vi "nanocal frontend server 18.vi"() -> ()   [LabVIEW 2018]
uses:
  nanocal/Nanocalorimetry/data/NanoCalLib.lvlibp/NanoReadings/NanoReadings_Parameters_TypeDef.ctl
  nanocal/Nanocalorimetry/data/NanoCalLib.lvlibp/NanoReadings/NanoReadings_Power.ctl
  nanocal/Nanocalorimetry/data/NanoCalLib.lvlibp/NanoReadings/NanoReadings_CandK.ctl
  nanocal/Nanocalorimetry/data/NanoCalLib.lvlibp/NanoReadings/NanoReadings_IandV.ctl
  nanocal/Nanocalorimetry/data/NanoCalLib.lvlibp/NanoReadings/NanoReadings_TdcTac.ctl
  nanocal/Nanocalorimetry/data/NanoCalLib.lvlibp/NanoReadings/NanoReadings_Phases.ctl
  nanocal/Nanocalorimetry/data/NanoCalLib.lvlibp/NanoReadings/NanoReadings_Frequencies.ctl
  nanocal/Nanocalorimetry/data/NanoCalLib.lvlibp/NanoReadings/NanoReadings_FirstHarmonic.ctl
  nanocal/Nanocalorimetry/data/NanoCalLib.lvlibp/NanoReadings/NanoReadings_Output.ctl
  nanocal/Nanocalorimetry/data/NanoCalLib.lvlibp/NanoReadings/NanoReadings_MagneticFieldEtc.ctl
  nanocal/Nanocalorimetry/data/NanoCalLib.lvlibp/NanoReadings/NanoReadings_Calibration.ctl
  nanocal/Nanocalorimetry/data/NanoCalLib.lvlibp/NanoReadings/NanoReadings_CTetc.ctl
  nanocal/Nanocalorimetry/data/NanoCalLib.lvlibp/NanoReadings/NanoReadings_2ndHarmonic.ctl
  nanocal/Nanocalorimetry/data/NanoCalLib.lvlibp/NanoReadings/NanoReadings_Resistance.ctl
  nanocal/Nanocalorimetry/data/NanoCalLib.lvlibp/NanoReadings/NanoReadings_TimeEtc.ctl
  frontend -- data type.ctl
  nanocal/Nanocalorimetry/data/NanoCalLib.lvlibp
  nanocal/Nanocalorimetry/data/NanoCalLib.lvlibp/NanoReadings/NanoReadings.lvlib
panel:
  in  "Latest data 2":T1={"Power"={"PHs (W)"=0.0, "PHr (W)"=0.0, "Ps,dc (W)"=0.0, "Pr,dc (W)"=0.0, "PHs,dc (W)"=0.0, "PHr,dc (W)"=0.0, "Ps,ac (W)"=0.0, "Pr,ac (W)"=0.0, "PHs/PHr"=0.0, "Poffs (W)"=0.0, "Ps total (W)"=0.0, "Pr total (W)"=0.0, "Ps-Pr total (W)"=0.0, "Ps,offs (W)"=0.0}, "C and K"={"Cs (J/K)"=0.0, "Ks (W/K)"=0.0, "Cr (J/K)"=0.0, "Kr (W/K)"=0.0, "Cdiff (J/K)"=0.0, "Cs-Cr (J/K)"=0.0, "Cdiff old style (J/K)"=0.0, "Cr from S,diff (J/K)"=0.0}, "IV dc"={"Is,dc (A)"=0.0, "Ir,dc (A)"=0.0, "Us,dc (V)"=0.0, "Ur,dc (V)"=0.0, "Udiff,dc (V)"=0.0, "IHs dc (A)"=0.0, "UHs dc (V)"=0.0, "IHr dc (A)"=0.0, "UHr dc (V)"=0.0, "Uoffs dc (V)"=0.0, "Ioffs dc (A)"=0.0}, "Tdc,Tac"={"Ts (K)"=0.0, "Tr (K)"=0.0, "Tdiff from Rs,Rr"=0.0, "Tdiff from Udiff (K)"=0.0, "Ts,ac (K)"=0.0, "Tr,ac (K)"=0.0, "Tdiff,ac (K)"=0.0, "Ts,ac driftcorr (K)"=0.0, "Tr,ac driftcorr (K)"=0.0, "Tr,ac from Ts,diff,ac (K)"=0.0, "T target (K)"=0.0}, "Phases"={"Phi Is (deg)"=0.0, "Phi Us (deg)"=0.0, "Phi Ir (deg)"=0.0, "Phi Ur (deg)"=0.0, "Phi Udiff (deg)"=0.0, "Phi IHs (deg)"=0.0, "Phi UHs (deg)"=0.0, "Phi IHr (deg)"=0.0, "Phi UHr (deg)"=0.0, "Phi R from S,diff (deg)"=0.0, "Phi Is 1st (deg)"=0.0, "Phi Us 1st (deg)"=0.0, "Phi Ir 1st (deg)"=0.0, "Phi Ur 1st (deg)"=0.0, "Phi Udiff 1st (deg)"=0.0, "Phi Udiff, raw (deg)"=0.0}, "f etc"={"f (Hz)"=36.0, "f therm (Hz)"=0.0, "omega (rad/s)"=0.0, "Tan Phi S/diff"=0.0, "Sin Phi"=0.0, "Cos Phi"=0.0, "f mix (Hz)"=0.0, "tau (s)"=0.0}, "IV 1st harm"={"Is,ac 1st (A)"=0.0, "Ir,ac 1st (A)"=0.0, "Us,ac 1st (V)"=0.0, "Ur,ac 1st (V)"=0.0, "Udiff,ac 1st (V)"=0.0, "IHs (A)"=0.0, "UHs (V)"=0.0, "IHr (A)"=0.0, "UHr (V)"=0.0}, "ForAveraging"={"SinTherm"=[], "CosTherm"=[], "SinHeats"=[], "CosHeats"=[]}, "Output"={"S phase (deg)"=0.0, "R phase (deg)"=0.0, "Hs ac out (Vrms)"=0.0, "Hr ac out (Vrms)"=0.0, "S Therm dc out (V)"=0.0, "R Therm dc out (V)"=0.0, "S Therm ac out (Vrms)"=0.0, "R Therm ac out (Vrms)"=0.0, "Offset dc out (V)"=0.0, "Hs dc out (V)"=0.0, "Hr dc out (V)"=0.0, "Offset ac out (Vrms)"=0.0}, "Magnetic field etc."={"H (T)"=0.0, "T probe (K)"=0.0, "Polar angle (deg)"=0.0, "Azimuthal angle (deg)"=0.0}, "Calibration"={"1+Rs/RIs factor"=0.0, "1+RIs/Rs factor"=0.0, "Rs,scaled (ohm)"=0.0, "Rr,scaled (ohm)"=0.0, "R lead S (ohm)"=0.0, "R lead R (ohm)"=0.0, "|dlnR/dlnT| S"=0.0, "|dlnR/dlnT| R"=0.0, "dTs/dt (mK/s)"=0.0, "dTr/dt (mK/s)"=0.0}, "CT etc"={"Cs/T (J/K^2)"=5.0, "Cr/T (J/K^2)"=0.0, "Cdiff/T (J/K^2)"=0.0, "(Cs-Cr)/T (J/K^2)"=0.0, "Cdiff/T old style (J/K^2)"=0.0, "Cr/T from S,diff (J/K^2)"=0.0, "Ts^2 (K^2)"=3.0, "Tr^2 (K^2)"=0.0}, "IV 2nd harm"={"Is,ac (A)"=0.0, "Ir,ac (A)"=0.0, "Us,ac (V)"=0.0, "Ur,ac (V)"=0.0, "Udiff,ac (V)"=0.0}, "Resistance"={"RHs (ohm)"=0.0, "RHr (ohm)"=0.0, "Rs (ohm)"=0.0, "Rr (ohm)"=0.0, "RHs,dc (ohm)"=0.0, "RHr,dc (ohm)"=0.0, "Rs,ac (ohm)"=0.0, "Rr,ac (ohm)"=0.0, "Roffs (ohm)"=0.0}, "Time etc"={"Time (s)"=0.0, "Datapoint index"=0.0, "Datapoint time (s)"=0.0}} {"Time etc"."Datapoint time (s)" format="%#_7g"; "Time etc"."Datapoint index" format="%#_7g"; "Time etc"."Time (s)" format="%#_7g"; "Resistance"."Roffs (ohm)" format="%#_7g"; "Resistance"."Rr,ac (ohm)" format="%#_7g"; "Resistance"."Rs,ac (ohm)" format="%#_7g"; "Resistance"."RHr,dc (ohm)" format="%#_7g"; "Resistance"."RHs,dc (ohm)" format="%#_7g"; "Resistance"."Rr (ohm)" format="%#_7g"; "Resistance"."Rs (ohm)" format="%#_7g"; "Resistance"."RHr (ohm)" format="%#_7g"; "Resistance"."RHs (ohm)" format="%#_7g"; "IV 2nd harm"."Udiff,ac (V)" format="%#_7g"; "IV 2nd harm"."Ur,ac (V)" format="%#_7g"; "IV 2nd harm"."Us,ac (V)" format="%#_7g"; "IV 2nd harm"."Ir,ac (A)" format="%#_7g"; "IV 2nd harm"."Is,ac (A)" format="%#_7g"; "CT etc"."Tr^2 (K^2)" format="%#_7g"; "CT etc"."Ts^2 (K^2)" format="%#_7g"; "Calibration"."dTr/dt (mK/s)" format="%#_7g"; "Calibration"."dTs/dt (mK/s)" format="%#_7g"; "Output"."Hr dc out (V)" min=0.0 max=7.0707; "Output"."Hs dc out (V)" min=0.0 max=7.0707; "Output"."Hr ac out (Vrms)" min=0.0 max=7.0707; "Output"."Hs ac out (Vrms)" min=0.0 max=7.0707; "Output"."R phase (deg)" format="%#_7g"; "Output"."S phase (deg)" format="%#_7g"; "IV 1st harm"."UHr (V)" format="%#_7g"; "IV 1st harm"."IHr (A)" format="%#_7g"; "IV 1st harm"."UHs (V)" format="%#_7g"; "IV 1st harm"."IHs (A)" format="%#_7g"; "IV 1st harm"."Udiff,ac 1st (V)" format="%#_7g"; "IV 1st harm"."Ur,ac 1st (V)" format="%#_7g"; "IV 1st harm"."Us,ac 1st (V)" format="%#_7g"; "IV 1st harm"."Ir,ac 1st (A)" format="%#_7g"; "IV 1st harm"."Is,ac 1st (A)" format="%#_7g"; "f etc"."tau (s)" format="%#_7g"; "f etc"."Cos Phi" format="%#_7g"; "f etc"."Sin Phi" format="%#_7g"; "f etc"."Tan Phi S/diff" format="%#_7g"; "Phases"."Phi Udiff, raw (deg)" format="%#_7g"; "Phases"."Phi Udiff 1st (deg)" format="%#_7g"; "Phases"."Phi Ur 1st (deg)" format="%#_7g"; "Phases"."Phi Ir 1st (deg)" format="%#_7g"; "Phases"."Phi Us 1st (deg)" format="%#_7g"; "Phases"."Phi Is 1st (deg)" format="%#_7g"; "Phases"."Phi R from S,diff (deg)" format="%#_7g"; "Phases"."Phi UHr (deg)" format="%#_7g"; "Phases"."Phi IHr (deg)" format="%#_7g"; "Phases"."Phi UHs (deg)" format="%#_7g"; "Phases"."Phi IHs (deg)" format="%#_7g"; "Phases"."Phi Udiff (deg)" format="%#_7g"; "Phases"."Phi Ur (deg)" format="%#_7g"; "Phases"."Phi Ir (deg)" format="%#_7g"; "Phases"."Phi Us (deg)" format="%#_7g"; "Phases"."Phi Is (deg)" format="%#_7g"; "Tdc,Tac"."T target (K)" format="%#_7g"; "Tdc,Tac"."Tr,ac from Ts,diff,ac (K)" format="%#_7g"; "Tdc,Tac"."Tr,ac driftcorr (K)" format="%#_7g"; "Tdc,Tac"."Ts,ac driftcorr (K)" format="%#_7g"; "Tdc,Tac"."Tdiff,ac (K)" format="%#_7g"; "Tdc,Tac"."Tr,ac (K)" format="%#_7g"; "Tdc,Tac"."Ts,ac (K)" format="%#_7g"; "Tdc,Tac"."Tdiff from Udiff (K)" format="%#_7g"; "Tdc,Tac"."Tdiff from Rs,Rr" format="%#_7g"; "Tdc,Tac"."Tr (K)" format="%#_7g"; "Tdc,Tac"."Ts (K)" format="%#_7g"; "IV dc"."Ioffs dc (A)" format="%#_7g"; "IV dc"."Uoffs dc (V)" format="%#_7g"; "IV dc"."UHr dc (V)" format="%#_7g"; "IV dc"."IHr dc (A)" format="%#_7g"; "IV dc"."UHs dc (V)" format="%#_7g"; "IV dc"."IHs dc (A)" format="%#_7g"; "IV dc"."Udiff,dc (V)" format="%#_7g"; "IV dc"."Ur,dc (V)" format="%#_7g"; "IV dc"."Us,dc (V)" format="%#_7g"; "IV dc"."Ir,dc (A)" format="%#_7g"; "IV dc"."Is,dc (A)" format="%#_7g"; "Power"."Ps,offs (W)" format="%#_7g"; "Power"."Ps-Pr total (W)" format="%#_7g"; "Power"."Pr total (W)" format="%#_7g"; "Power"."Ps total (W)" format="%#_7g"; "Power"."Poffs (W)" format="%#_7g"; "Power"."PHs/PHr" format="%#_7g"; "Power"."Pr,ac (W)" format="%#_7g"; "Power"."Ps,ac (W)" format="%#_7g"; "Power"."PHr,dc (W)" format="%#_7g"; "Power"."PHs,dc (W)" format="%#_7g"; "Power"."Pr,dc (W)" format="%#_7g"; "Power"."Ps,dc (W)" format="%#_7g"; "Power"."PHr (W)" format="%#_7g"; "Power"."PHs (W)" format="%#_7g"}
  out "Numeric":i32=90
  out "output cluster":T16
  in  "milliseconds to wait":u32=100
  in  "Stop":bool
  out "Latest data":T1 {"Time etc"."Datapoint time (s)" format="%#_7g"; "Time etc"."Datapoint index" format="%#_7g"; "Time etc"."Time (s)" format="%#_7g"; "Resistance"."Roffs (ohm)" format="%#_7g"; "Resistance"."Rr,ac (ohm)" format="%#_7g"; "Resistance"."Rs,ac (ohm)" format="%#_7g"; "Resistance"."RHr,dc (ohm)" format="%#_7g"; "Resistance"."RHs,dc (ohm)" format="%#_7g"; "Resistance"."Rr (ohm)" format="%#_7g"; "Resistance"."Rs (ohm)" format="%#_7g"; "Resistance"."RHr (ohm)" format="%#_7g"; "Resistance"."RHs (ohm)" format="%#_7g"; "IV 2nd harm"."Udiff,ac (V)" format="%#_7g"; "IV 2nd harm"."Ur,ac (V)" format="%#_7g"; "IV 2nd harm"."Us,ac (V)" format="%#_7g"; "IV 2nd harm"."Ir,ac (A)" format="%#_7g"; "IV 2nd harm"."Is,ac (A)" format="%#_7g"; "CT etc"."Tr^2 (K^2)" format="%#_7g"; "CT etc"."Ts^2 (K^2)" format="%#_7g"; "Calibration"."dTr/dt (mK/s)" format="%#_7g"; "Calibration"."dTs/dt (mK/s)" format="%#_7g"; "Output"."Hr dc out (V)" min=0.0 max=7.0707; "Output"."Hs dc out (V)" min=0.0 max=7.0707; "Output"."Hr ac out (Vrms)" min=0.0 max=7.0707; "Output"."Hs ac out (Vrms)" min=0.0 max=7.0707; "Output"."R phase (deg)" format="%#_7g"; "Output"."S phase (deg)" format="%#_7g"; "IV 1st harm"."UHr (V)" format="%#_7g"; "IV 1st harm"."IHr (A)" format="%#_7g"; "IV 1st harm"."UHs (V)" format="%#_7g"; "IV 1st harm"."IHs (A)" format="%#_7g"; "IV 1st harm"."Udiff,ac 1st (V)" format="%#_7g"; "IV 1st harm"."Ur,ac 1st (V)" format="%#_7g"; "IV 1st harm"."Us,ac 1st (V)" format="%#_7g"; "IV 1st harm"."Ir,ac 1st (A)" format="%#_7g"; "IV 1st harm"."Is,ac 1st (A)" format="%#_7g"; "f etc"."tau (s)" format="%#_7g"; "f etc"."Cos Phi" format="%#_7g"; "f etc"."Sin Phi" format="%#_7g"; "f etc"."Tan Phi S/diff" format="%#_7g"; "Phases"."Phi Udiff, raw (deg)" format="%#_7g"; "Phases"."Phi Udiff 1st (deg)" format="%#_7g"; "Phases"."Phi Ur 1st (deg)" format="%#_7g"; "Phases"."Phi Ir 1st (deg)" format="%#_7g"; "Phases"."Phi Us 1st (deg)" format="%#_7g"; "Phases"."Phi Is 1st (deg)" format="%#_7g"; "Phases"."Phi R from S,diff (deg)" format="%#_7g"; "Phases"."Phi UHr (deg)" format="%#_7g"; "Phases"."Phi IHr (deg)" format="%#_7g"; "Phases"."Phi UHs (deg)" format="%#_7g"; "Phases"."Phi IHs (deg)" format="%#_7g"; "Phases"."Phi Udiff (deg)" format="%#_7g"; "Phases"."Phi Ur (deg)" format="%#_7g"; "Phases"."Phi Ir (deg)" format="%#_7g"; "Phases"."Phi Us (deg)" format="%#_7g"; "Phases"."Phi Is (deg)" format="%#_7g"; "Tdc,Tac"."T target (K)" format="%#_7g"; "Tdc,Tac"."Tr,ac from Ts,diff,ac (K)" format="%#_7g"; "Tdc,Tac"."Tr,ac driftcorr (K)" format="%#_7g"; "Tdc,Tac"."Ts,ac driftcorr (K)" format="%#_7g"; "Tdc,Tac"."Tdiff,ac (K)" format="%#_7g"; "Tdc,Tac"."Tr,ac (K)" format="%#_7g"; "Tdc,Tac"."Ts,ac (K)" format="%#_7g"; "Tdc,Tac"."Tdiff from Udiff (K)" format="%#_7g"; "Tdc,Tac"."Tdiff from Rs,Rr" format="%#_7g"; "Tdc,Tac"."Tr (K)" format="%#_7g"; "Tdc,Tac"."Ts (K)" format="%#_7g"; "IV dc"."Ioffs dc (A)" format="%#_7g"; "IV dc"."Uoffs dc (V)" format="%#_7g"; "IV dc"."UHr dc (V)" format="%#_7g"; "IV dc"."IHr dc (A)" format="%#_7g"; "IV dc"."UHs dc (V)" format="%#_7g"; "IV dc"."IHs dc (A)" format="%#_7g"; "IV dc"."Udiff,dc (V)" format="%#_7g"; "IV dc"."Ur,dc (V)" format="%#_7g"; "IV dc"."Us,dc (V)" format="%#_7g"; "IV dc"."Ir,dc (A)" format="%#_7g"; "IV dc"."Is,dc (A)" format="%#_7g"; "Power"."Ps,offs (W)" format="%#_7g"; "Power"."Ps-Pr total (W)" format="%#_7g"; "Power"."Pr total (W)" format="%#_7g"; "Power"."Ps total (W)" format="%#_7g"; "Power"."Poffs (W)" format="%#_7g"; "Power"."PHs/PHr" format="%#_7g"; "Power"."Pr,ac (W)" format="%#_7g"; "Power"."Ps,ac (W)" format="%#_7g"; "Power"."PHr,dc (W)" format="%#_7g"; "Power"."PHs,dc (W)" format="%#_7g"; "Power"."Pr,dc (W)" format="%#_7g"; "Power"."Ps,dc (W)" format="%#_7g"; "Power"."PHr (W)" format="%#_7g"; "Power"."PHs (W)" format="%#_7g"}
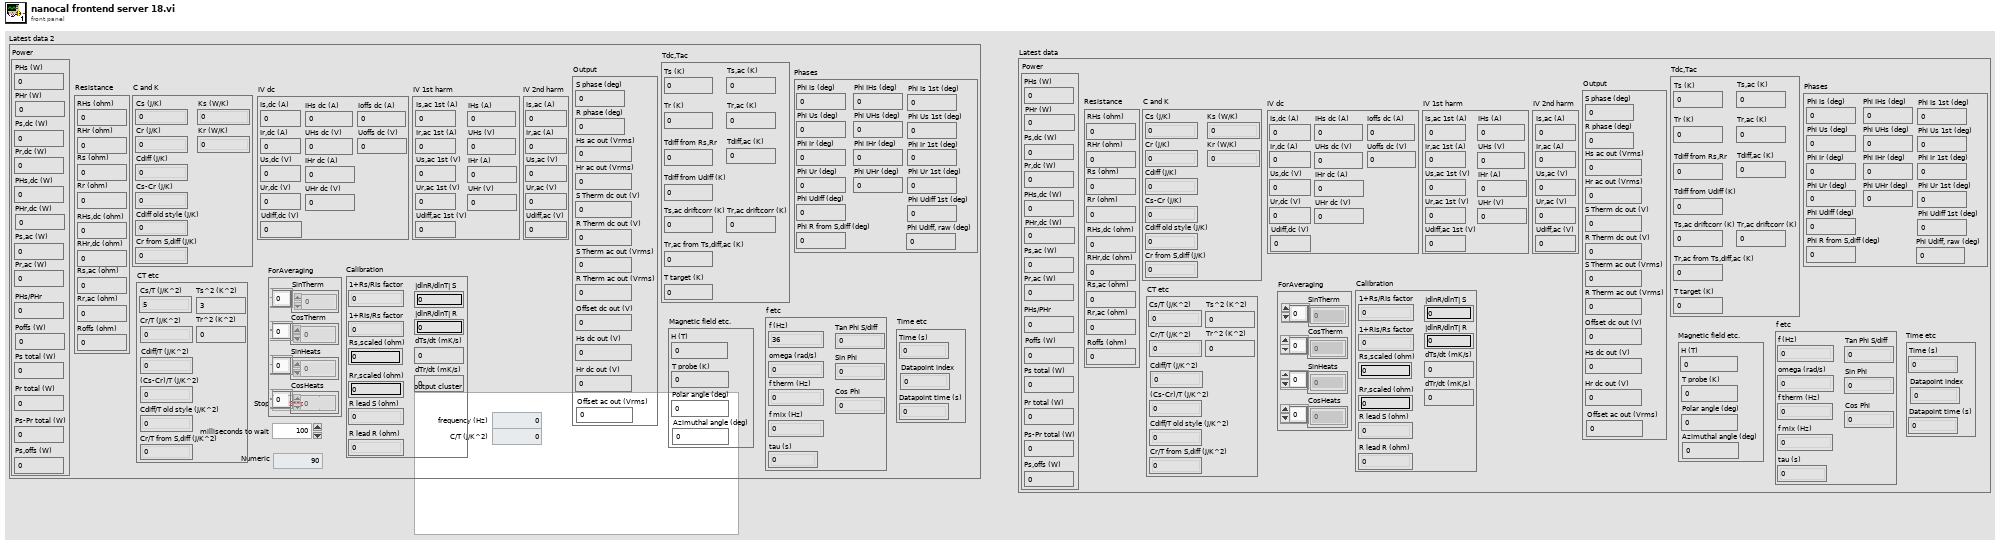
[diagram p1: front panel]
types:
  T1 = typedef "NanoCalLib.lvlibp/NanoReadings.lvlib/NanoReadings_Parameters_TypeDef.ctl" = cluster{"Power":T2, "C and K":T3, "IV dc":T4, "Tdc,Tac":T5, "Phases":T6, "f etc":T7, "IV 1st harm":T8, "ForAveraging":cluster{"SinTherm":dbl[], "CosTherm":dbl[], "SinHeats":dbl[], "CosHeats":dbl[]}, "Output":T9, "Magnetic field etc.":T10, "Calibration":T11, "CT etc":T12, "IV 2nd harm":T13, "Resistance":T14, "Time etc":T15}
  T2 = typedef "NanoCalLib.lvlibp/NanoReadings.lvlib/NanoReadings_Power.ctl" = cluster{"PHs (W)":dbl, "PHr (W)":dbl, "Ps,dc (W)":dbl, "Pr,dc (W)":dbl, "PHs,dc (W)":dbl, "PHr,dc (W)":dbl, "Ps,ac (W)":dbl, "Pr,ac (W)":dbl, "PHs/PHr":dbl, "Poffs (W)":dbl, "Ps total (W)":dbl, "Pr total (W)":dbl, "Ps-Pr total (W)":dbl, "Ps,offs (W)":dbl}
  T3 = typedef "NanoCalLib.lvlibp/NanoReadings.lvlib/NanoReadings_CandK.ctl" = cluster{"Cs (J/K)":dbl, "Ks (W/K)":dbl, "Cr (J/K)":dbl, "Kr (W/K)":dbl, "Cdiff (J/K)":dbl, "Cs-Cr (J/K)":dbl, "Cdiff old style (J/K)":dbl, "Cr from S,diff (J/K)":dbl}
  T4 = typedef "NanoCalLib.lvlibp/NanoReadings.lvlib/NanoReadings_IandV.ctl" = cluster{"Is,dc (A)":dbl, "Ir,dc (A)":dbl, "Us,dc (V)":dbl, "Ur,dc (V)":dbl, "Udiff,dc (V)":dbl, "IHs dc (A)":dbl, "UHs dc (V)":dbl, "IHr dc (A)":dbl, "UHr dc (V)":dbl, "Uoffs dc (V)":dbl, "Ioffs dc (A)":dbl}
  T5 = typedef "NanoCalLib.lvlibp/NanoReadings.lvlib/NanoReadings_TdcTac.ctl" = cluster{"Ts (K)":dbl, "Tr (K)":dbl, "Tdiff from Rs,Rr":dbl, "Tdiff from Udiff (K)":dbl, "Ts,ac (K)":dbl, "Tr,ac (K)":dbl, "Tdiff,ac (K)":dbl, "Ts,ac driftcorr (K)":dbl, "Tr,ac driftcorr (K)":dbl, "Tr,ac from Ts,diff,ac (K)":dbl, "T target (K)":dbl}
  T6 = typedef "NanoCalLib.lvlibp/NanoReadings.lvlib/NanoReadings_Phases.ctl" = cluster{"Phi Is (deg)":dbl, "Phi Us (deg)":dbl, "Phi Ir (deg)":dbl, "Phi Ur (deg)":dbl, "Phi Udiff (deg)":dbl, "Phi IHs (deg)":dbl, "Phi UHs (deg)":dbl, "Phi IHr (deg)":dbl, "Phi UHr (deg)":dbl, "Phi R from S,diff (deg)":dbl, "Phi Is 1st (deg)":dbl, "Phi Us 1st (deg)":dbl, "Phi Ir 1st (deg)":dbl, "Phi Ur 1st (deg)":dbl, "Phi Udiff 1st (deg)":dbl, "Phi Udiff, raw (deg)":dbl}
  T7 = typedef "NanoCalLib.lvlibp/NanoReadings.lvlib/NanoReadings_Frequencies.ctl" = cluster{"f (Hz)":dbl, "f therm (Hz)":dbl, "omega (rad/s)":dbl, "Tan Phi S/diff":dbl, "Sin Phi":dbl, "Cos Phi":dbl, "f mix (Hz)":dbl, "tau (s)":dbl}
  T8 = typedef "NanoCalLib.lvlibp/NanoReadings.lvlib/NanoReadings_FirstHarmonic.ctl" = cluster{"Is,ac 1st (A)":dbl, "Ir,ac 1st (A)":dbl, "Us,ac 1st (V)":dbl, "Ur,ac 1st (V)":dbl, "Udiff,ac 1st (V)":dbl, "IHs (A)":dbl, "UHs (V)":dbl, "IHr (A)":dbl, "UHr (V)":dbl}
  T9 = typedef "NanoCalLib.lvlibp/NanoReadings.lvlib/NanoReadings_Output.ctl" = cluster{"S phase (deg)":dbl, "R phase (deg)":dbl, "Hs ac out (Vrms)":dbl, "Hr ac out (Vrms)":dbl, "S Therm dc out (V)":dbl, "R Therm dc out (V)":dbl, "S Therm ac out (Vrms)":dbl, "R Therm ac out (Vrms)":dbl, "Offset dc out (V)":dbl, "Hs dc out (V)":dbl, "Hr dc out (V)":dbl, "Offset ac out (Vrms)":dbl}
  T10 = typedef "NanoCalLib.lvlibp/NanoReadings.lvlib/NanoReadings_MagneticFieldEtc.ctl" = cluster{"H (T)":dbl, "T probe (K)":dbl, "Polar angle (deg)":dbl, "Azimuthal angle (deg)":dbl}
  T11 = typedef "NanoCalLib.lvlibp/NanoReadings.lvlib/NanoReadings_Calibration.ctl" = cluster{"1+Rs/RIs factor":dbl, "1+RIs/Rs factor":dbl, "Rs,scaled (ohm)":dbl, "Rr,scaled (ohm)":dbl, "R lead S (ohm)":dbl, "R lead R (ohm)":dbl, "|dlnR/dlnT| S":dbl, "|dlnR/dlnT| R":dbl, "dTs/dt (mK/s)":dbl, "dTr/dt (mK/s)":dbl}
  T12 = typedef "NanoCalLib.lvlibp/NanoReadings.lvlib/NanoReadings_CTetc.ctl" = cluster{"Cs/T (J/K^2)":dbl, "Cr/T (J/K^2)":dbl, "Cdiff/T (J/K^2)":dbl, "(Cs-Cr)/T (J/K^2)":dbl, "Cdiff/T old style (J/K^2)":dbl, "Cr/T from S,diff (J/K^2)":dbl, "Ts^2 (K^2)":dbl, "Tr^2 (K^2)":dbl}
  T13 = typedef "NanoCalLib.lvlibp/NanoReadings.lvlib/NanoReadings_2ndHarmonic.ctl" = cluster{"Is,ac (A)":dbl, "Ir,ac (A)":dbl, "Us,ac (V)":dbl, "Ur,ac (V)":dbl, "Udiff,ac (V)":dbl}
  T14 = typedef "NanoCalLib.lvlibp/NanoReadings.lvlib/NanoReadings_Resistance.ctl" = cluster{"RHs (ohm)":dbl, "RHr (ohm)":dbl, "Rs (ohm)":dbl, "Rr (ohm)":dbl, "RHs,dc (ohm)":dbl, "RHr,dc (ohm)":dbl, "Rs,ac (ohm)":dbl, "Rr,ac (ohm)":dbl, "Roffs (ohm)":dbl}
  T15 = typedef "NanoCalLib.lvlibp/NanoReadings.lvlib/NanoReadings_TimeEtc.ctl" = cluster{"Time (s)":dbl, "Datapoint index":dbl, "Datapoint time (s)":dbl}
  T16 = typedef "frontend -- data type.ctl" = cluster{"frequency (Hz)":dbl, "C/T (J/K^2)":dbl}
  T17 = typedef "MCL.lvlibp/MCL_DataRef.ctl" = refnum<vi>
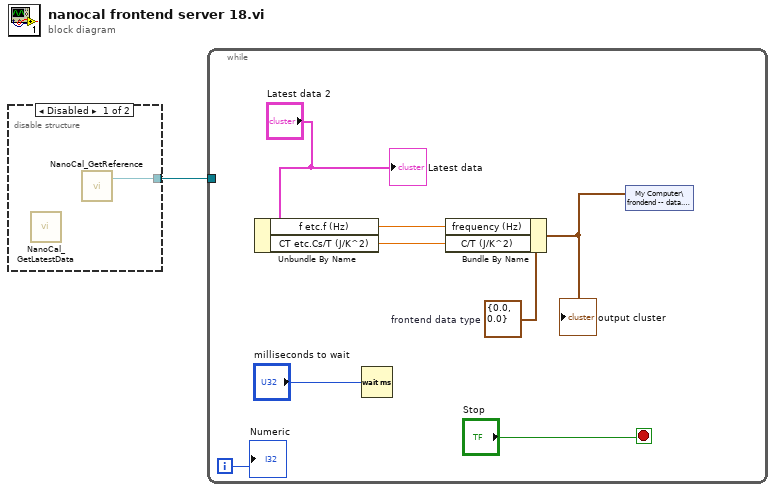
[diagram p0: block diagram]
diagram:
  n1 = disable-structure shown="Disabled" {
    disable-tunnel: [w2 _] -> w1
    frame Disabled {
      n2 = call "NanoCal_GetLatestData.vi"() -> ()  [unwired: 1 in, 1 out]
      n3 = call "NanoCal_GetReference.vi"() -> ("Connected MCL object"=w2:T17)  [unwired: 2 in, 1 out]
    }
    frame Enabled {
    }
  }
  n4 = while {
    tunnel: w1 -> [_]
    i -> [w4]
    stop <- "Stop" stop-if-true
    w8 = T16 {"frequency (Hz)"=0.0, "C/T (J/K^2)"=0.0}  # frontend data type
    n5 = Unbundle By Name("Latest data 2") -> ("f etc.f (Hz)"=w7:dbl, "CT etc.Cs/T (J/K^2)"=w6:dbl)
    n6 = Wait (ms)(milliseconds to wait="milliseconds to wait") -> ()  [unwired: 1 out]
    n7 = Bundle By Name(cluster=w8, "frequency (Hz)"=w7, "C/T (J/K^2)"=w6) -> (w5:T16)
    "output cluster" <- w5
    n8 = shared-variable "My Computer\\frondend -- data.lvlib\\data"(w5) -> ()  [unwired: 1 in, 1 out]
    "Latest data" <- "Latest data 2"
    "Numeric" <- w4
  }
